vi "RPC Method Template.vi"(8 "error in":errorcluster, 9 "ms timeout (10000)":i32=10000, 10 "Request Data":cluster{"Numeric":dbl}, 11 "gRPC Client in":refnum<class "Template Client.lvclass">) -> (0 "error out":errorcluster, 2 "Response Data":cluster{"Numeric":dbl}, 3 "gRPC Client out":refnum<class "Template Client.lvclass">)   [LabVIEW 2019, in "Template Client.lvlib" / "Template Client.lvclass"]
uses:
  Template Client.lvclass
  fa22ca14-33b2-4bc3-8699-3f27c9b27c9c.vi
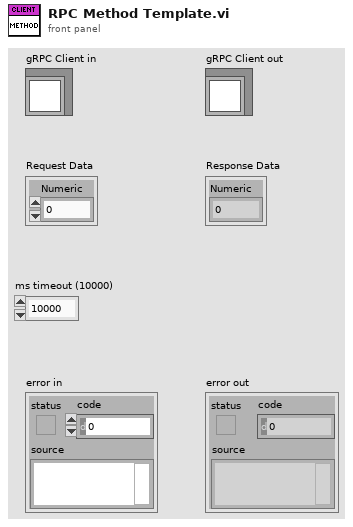
[diagram p1: front panel]
types:
  T1 = typedef "gprc-lvsupport-release.lvlib/grpcId.ctl" = u64
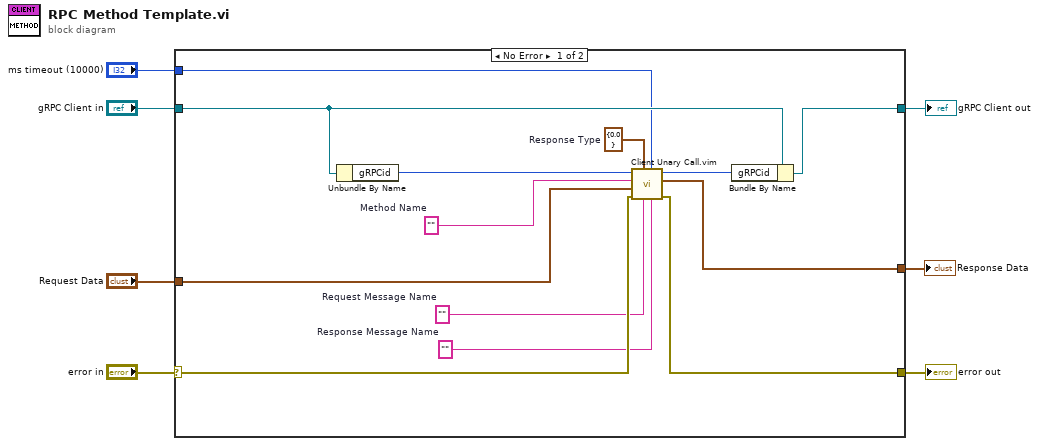
[diagram p0: block diagram]
diagram:
  n1 = case shown="No Error" "error in" {
    selector: "error in" -> [w16 w22]
    tunnel: [w15 w22] -> w6
    tunnel: [w17 w21] -> w4
    tunnel: "gRPC Client in" -> [w19 w21]
    tunnel: "Request Data" -> [w13 _]
    tunnel: [w12 _] -> w2
    tunnel: "ms timeout (10000)" -> [w8 _]
    frame No Error {
      w9 = ""  # Response Message Name
      w10 = ""  # Request Message Name
      w11 = cluster{"Numeric":dbl} {"Numeric"=0.0}  # Response Type
      w14 = ""  # Method Name
      n2 = Unbundle By Name(w19) -> ("gRPCid"=w20:T1)
      n3 = call "Client Unary Call.vim"("Response Message Name"=w9, "ms timeout (10000)"=w8, "Request Message Name"=w10, "Response Type"=w11, "error in"=w16, "Request Data"=w13, "Method Name"=w14, "ClientID in"=w20) -> ("error out"=w15:errorcluster, "Response Data"=w12:cluster{"Numeric":dbl}, "ClientID out"=w18:u64)  [unwired: 1 in]
      n4 = Bundle By Name(cluster=w19, "gRPCid"=w18) -> (w17:refnum<class "Template Client.lvclass">)
    }
    frame Error {
    }
  }
  "error out" <- w6
  "gRPC Client out" <- w4
  "Response Data" <- w2
